vi "Goto Degree.vi"(8 "Invert Motor":bool, 9 "Target Degrees":dbl, 10 "Input Degrees":dbl) -> (2 "Output Motor Speed":dbl)   [LabVIEW 2014]
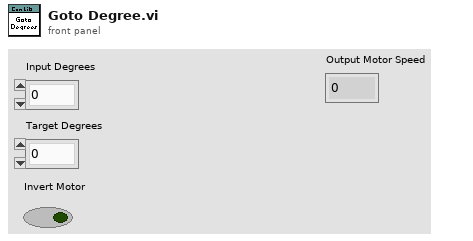
[diagram p1: front panel]
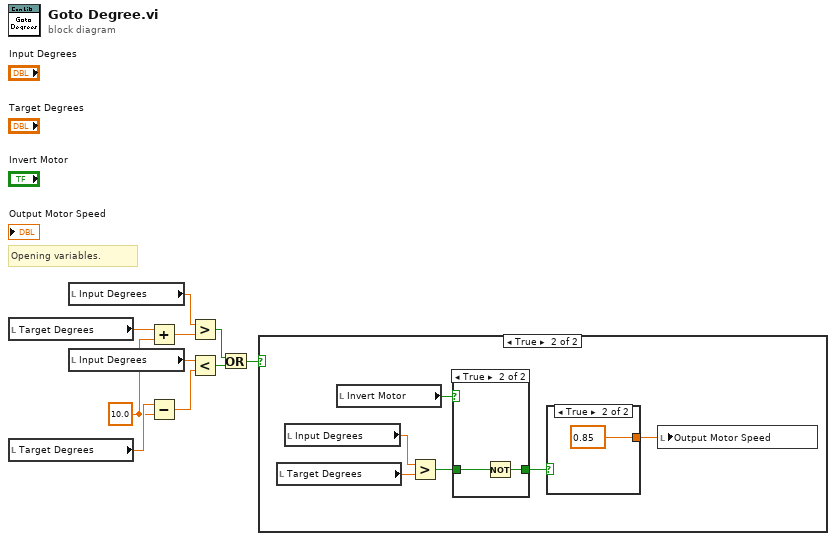
[diagram p0: block diagram]
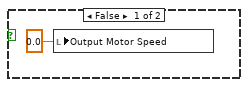
[diagram p2: hidden frame]
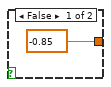
[diagram p3: hidden frame]
diagram:
  w3 = 10.0
  # "Opening variables."
  n1 = local read "Target Degrees"() -> (w8:dbl)
  n2 = local read "Target Degrees"() -> (w4:dbl)
  n3 = local read "Input Degrees"() -> (w10:dbl)
  n4 = local read "Input Degrees"() -> (w6:dbl)
  n5 = Add(x=w8, y=w3) -> (x+y=w9:dbl)
  n6 = Subtract(x=w4, y=w3) -> (x-y=w5:dbl)
  n7 = Greater?(x=w10, y=w9) -> (0:w7:bool)
  n8 = Less?(x=w6, y=w5) -> (x < y?=w2:bool)
  n9 = Or(x=w7, y=w2) -> (x .or. y?=w1:bool)
  n10 = case shown="True" w1 {
    frame False {
      n11 = local write "Output Motor Speed"(0.0) -> ()
    }
    frame True {
      n12 = local read "Target Degrees"() -> (w17:dbl)
      n13 = local read "Input Degrees"() -> (w16:dbl)
      n14 = local read "Invert Motor"() -> (w15:bool)
      n15 = Greater?(x=w16, y=w17) -> (0:w14:bool)
      n16 = case shown="True" w15 {
        tunnel: w14 -> [w20 w22]
        tunnel: [w20 w21] -> w13
        frame False {
        }
        frame True {
          n17 = Not(x=w22) -> (.not. x?=w21:bool)
        }
      }
      n18 = case shown="True" w13 {
        tunnel: [-0.85 0.85] -> w12
        frame False {
        }
        frame True {
        }
      }
      n19 = local write "Output Motor Speed"(w12) -> ()
    }
  }
